vi "System Read.vi"(8 "error in (no error)":errorcluster {"code" format="%.0x"}, 9 "Size":i32, 11 "instrument handle":refnum<k15>) -> (0 "error out":errorcluster {"code" format="%.0x"}, 1 "ActualSize":i32, 2 "Value":string, 3 "instrument handle out":refnum<k15>)   [LabVIEW 2014, in "Agilent NA.lvlib"]
doc: "This VI provides direct read access to the underlying instrument I/O interface."
uses:
  Agilent NA.lvlib
  AgNA.dll
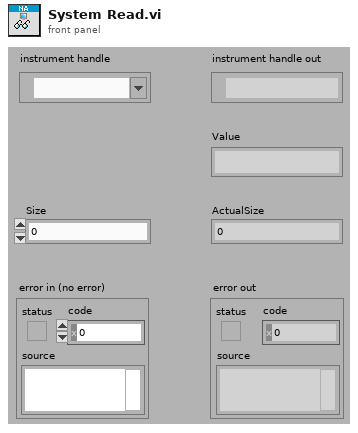
[diagram p1: front panel]
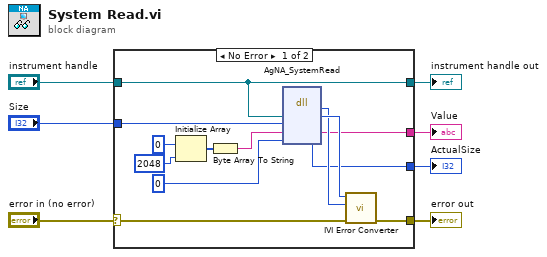
[diagram p0: block diagram]
diagram:
  n1 = case shown="No Error" "error in (no error)" {
    selector: "error in (no error)" -> [w18 w22]
    tunnel: [w17 w22] -> w7
    tunnel: "Size" -> [w16 _]
    tunnel: [w11 _] -> w4
    tunnel: [w9 _] -> w3
    tunnel: [w8 w21] -> w2
    tunnel: "instrument handle" -> [w8 w21]
    frame No Error {
      n2 = Initialize Array(u8 0 ("element"), 2048 ("dimension size")) -> (w14:u8[])
      n3 = Byte Array To String(unsigned byte array=w14) -> (string=w15:string)
      n4 = dll-call lib="AgNA**.dll" fn="AgNA_SystemRead"("Vi"=w8, "Size"=w16, "Value"=w15, "ActualSize"=0) -> (w19:i32, "Vi"=w20:u32, "Value"=w11:string, "ActualSize"=w9:i32)  [unwired: 4 in, 2 out]
      n5 = call "IVI Error Converter.vi"("error in (no error)"=w18, "IVI error code (0)"=w19, "instrument handle"=w20) -> ("error out"=w17:errorcluster)  [unwired: 7 in, 1 out]
    }
    frame Error {
    }
  }
  "error out" <- w7
  "instrument handle out" <- w2
  "Value" <- w4
  "ActualSize" <- w3
